vi "Write Hand.vi"(8 "error in (no error)":errorcluster, 10 "Hand":string, 11 "CardHand in":refnum<class "CardHand.lvclass">) -> (0 "error out":errorcluster, 3 "CardHand out":refnum<class "CardHand.lvclass">)   [LabVIEW 2021, in "2023.lvlib" / "CardHand.lvclass"]
uses:
  CardHand.lvclass
  CardHand.lvclass/CardHand.ctl
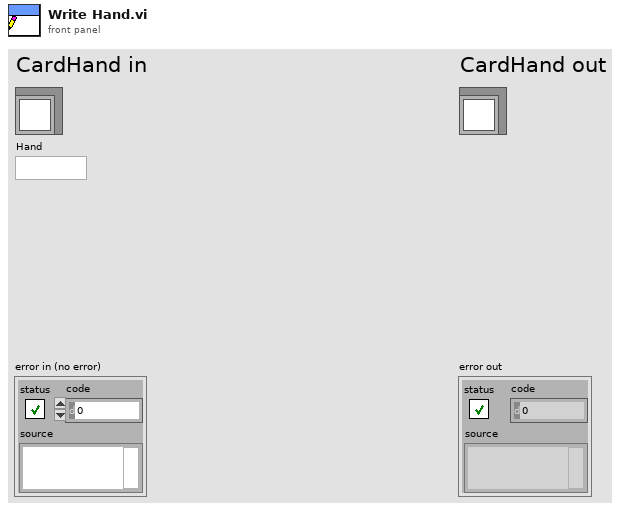
[diagram p1: front panel]
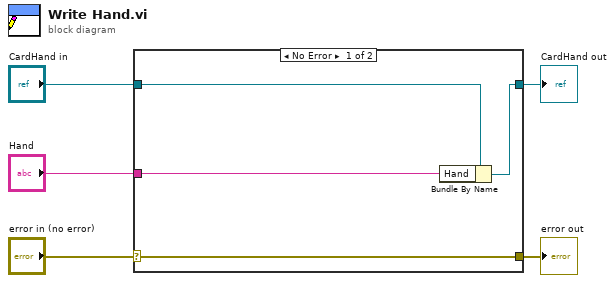
[diagram p0: block diagram]
diagram:
  n1 = case shown="No Error" "error in (no error)" {
    selector: "error in (no error)" -> [w9 w10]
    tunnel: [w9 w10] -> w4
    tunnel: [w7 w11] -> w2
    tunnel: "CardHand in" -> [w8 w11]
    tunnel: "Hand" -> [w6 _]
    frame No Error {
      n2 = Bundle By Name(cluster=w8, "Hand"=w6) -> (w7:refnum<class "CardHand.lvclass">)
    }
    frame Error {
    }
  }
  "error out" <- w4
  "CardHand out" <- w2
